vi "Archiver.Delete.vi"(8 "error in":errorcluster, 10 "files to remove":path[](array[path])) -> (0 "error out":errorcluster, 2 "last delete element":string)   [LabVIEW 2016]
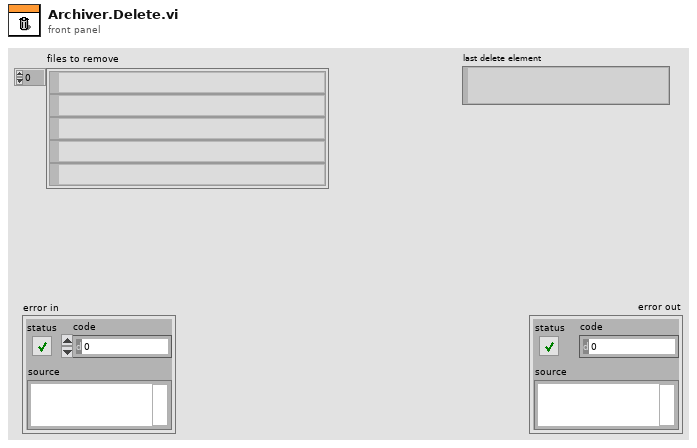
[diagram p1: front panel]
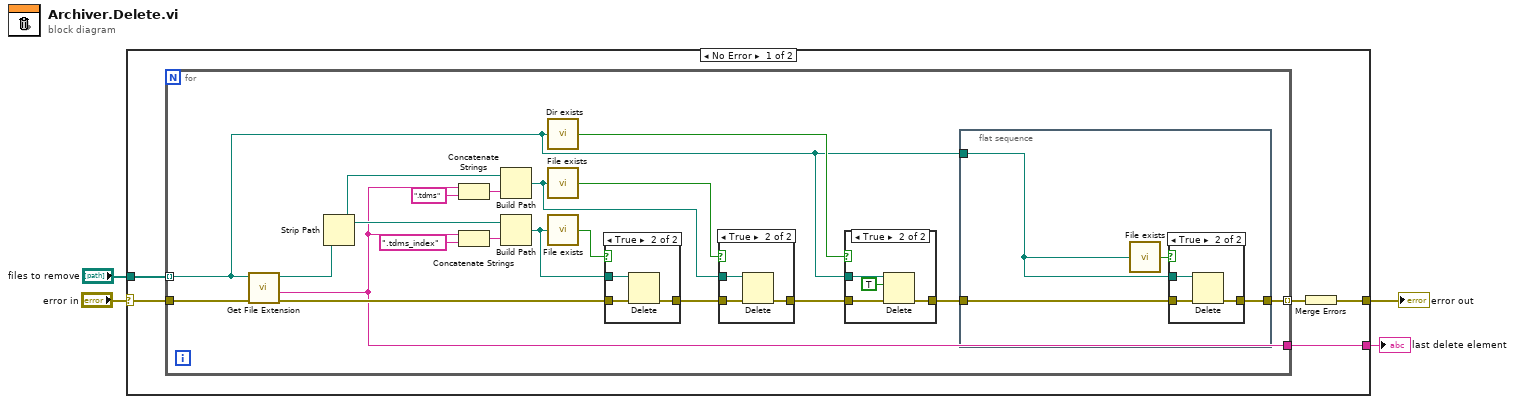
[diagram p0: block diagram]
diagram:
  n1 = case shown="No Error" "error in" {
    selector: "error in" -> [w9 w50]
    tunnel: [w6 w50] -> w4
    tunnel: "files to remove" -> [w8 _]
    tunnel: [w5 _] -> w1
    frame No Error {
      n2 = for {
        tunnel: w8 -> [w13] mode=indexing
        tunnel: w9 -> [w24]
        tunnel: [w11] -> w7 mode=indexing
        tunnel: [w10] -> w5
        n3 = call <vilib>:"Get File Extension.vi"("error in (no error)"=w24, "file"=w13) -> ("error out"=w19:errorcluster, "filename without extension"=w10:string, "dup file"=w18:path)  [unwired: 5 in, 2 out]
        n4 = Strip Path(path=w18) -> (stripped path=w15:path)  [unwired: 1 out]
        n5 = Concatenate Strings(w10, ".tdms" ("string")) -> (w16:string)
        n6 = Concatenate Strings(w10, ".tdms_index" ("string")) -> (w28:string)
        n7 = Build Path(base path=w15, name or relative path=w16) -> (appended path=w14:path)
        n8 = Build Path(base path=w15, name or relative path=w28) -> (appended path=w26:path)
        n9 = call "Dir exists.vi"("dir path"=w13) -> ("exists?"=w21:bool)  [unwired: 4 in]
        n10 = call "File exists.vi"("file path"=w14) -> ("exists?"=w22:bool)  [unwired: 4 in]
        n11 = call "File exists.vi"("file path"=w26) -> ("exists?"=w23:bool)  [unwired: 4 in]
        n12 = case shown="True" w23 {
          tunnel: w19 -> [w42 w45]
          tunnel: w26 -> [_ w44]
          tunnel: [w42 w43] -> w25
          frame False {
          }
          frame True {
            n13 = Delete(path (use dialog)=w44, error in=w45) -> (error out=w43:errorcluster)  [unwired: 3 in, 2 out]
          }
        }
        n14 = case shown="True" w22 {
          tunnel: w25 -> [w46 w49]
          tunnel: w14 -> [_ w48]
          tunnel: [w46 w47] -> w20
          frame False {
          }
          frame True {
            n15 = Delete(path (use dialog)=w48, error in=w49) -> (error out=w47:errorcluster)  [unwired: 3 in, 2 out]
          }
        }
        n16 = case shown="True" w21 {
          tunnel: w20 -> [w37 w41]
          tunnel: w13 -> [_ w40]
          tunnel: [w37 w39] -> w12
          frame False {
          }
          frame True {
            n17 = Delete(path (use dialog)=w40, entire hierarchy (F)=TRUE, error in=w41) -> (error out=w39:errorcluster)  [unwired: 2 in, 2 out]
          }
        }
        n18 = flat-sequence {
          tunnel: w13 -> [w31]
          tunnel: w12 -> [w30]
          tunnel: [w29] -> w11
          frame #0 {
            n19 = call "File exists.vi"("file path"=w31) -> ("exists?"=w32:bool)  [unwired: 4 in]
            n20 = case shown="True" w32 {
              tunnel: w30 -> [w33 w36]
              tunnel: w31 -> [_ w35]
              tunnel: [w33 w34] -> w29
              frame False {
              }
              frame True {
                n21 = Delete(path (use dialog)=w35, error in=w36) -> (error out=w34:errorcluster)  [unwired: 3 in, 2 out]
              }
            }
          }
        }
      }
      n22 = Merge Errors(w7) -> (w6:errorcluster)
    }
    frame Error {
    }
  }
  "error out" <- w4
  "last delete element" <- w1
